vi "initializePIstages.vi"(0 "xy stage":bool=TRUE, 1 "z stage":bool=TRUE) -> (2 "XY stage":T2, 3 "Z stage":T1, 4 "current xPos (mm)":dbl, 5 "current yPos (mm)":dbl, 6 "current zPos (mm)":dbl)   [LabVIEW 2015]
panel:
  in  "Z stage":T1={"System no."=2, "zIdx"=1, "zLim (mm)"=13.0, "0, 1"=0} {"System no." min=1 step=1}
  in  "XY stage":T2={"System no."=1, "xIdx"=1, "yIdx"=2, "xLim (mm)"=67.5, "yLim (mm)"=42.5, "0, 1"=0} {"System no." min=1 step=1}
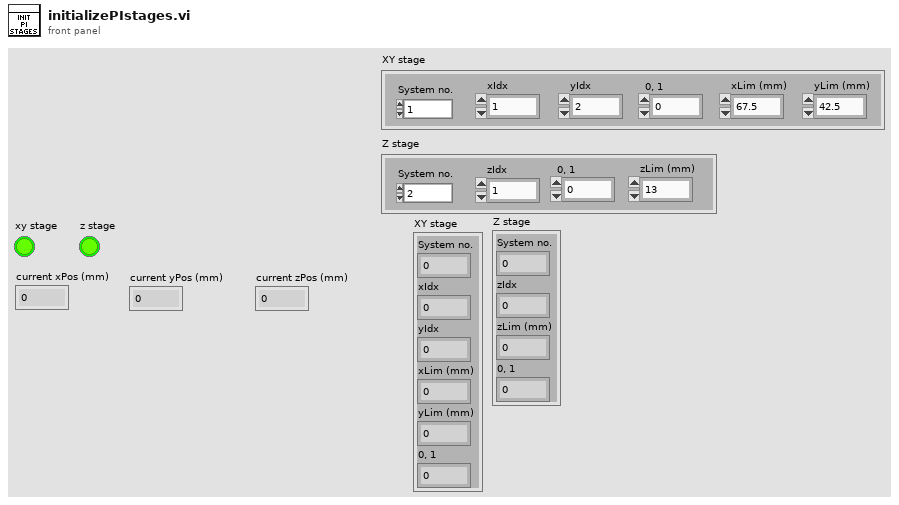
[diagram p1: front panel]
types:
  T1 = cluster{"System no.":i32, "zIdx":i32, "zLim (mm)":dbl, "0, 1":i16}
  T2 = cluster{"System no.":i32, "xIdx":i32, "yIdx":i32, "xLim (mm)":dbl, "yLim (mm)":dbl, "0, 1":i16}
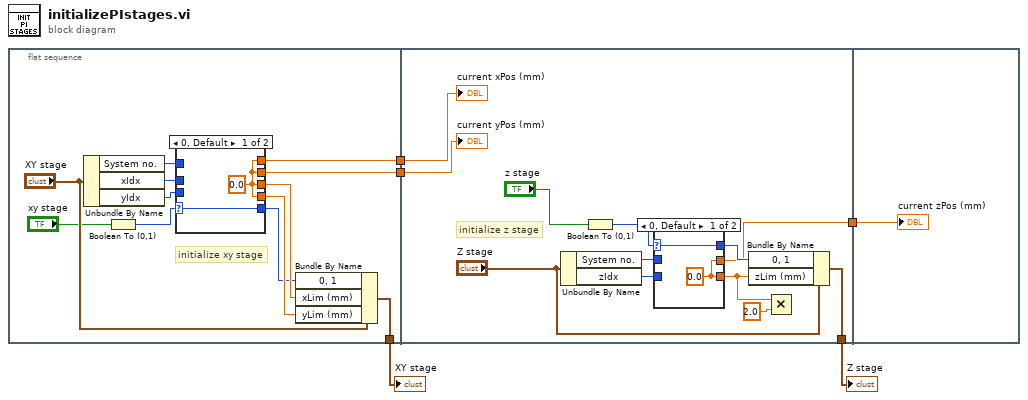
[diagram p0: block diagram]
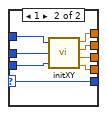
[diagram p2: hidden frame]
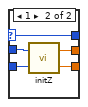
[diagram p3: hidden frame]
diagram:
  n1 = flat-sequence {
    tunnel: [w14] -> w5
    tunnel: [w13] -> w4
    tunnel: [w6] -> w2
    tunnel: w5 -> [w39]
    tunnel: w4 -> [w38]
    tunnel: [w32] -> w3
    tunnel: [w28] -> w1
    tunnel: w3 -> [w47]
    frame #0 {
      # "initialize xy stage"
      n2 = Unbundle By Name("XY stage") -> ("System no."=w17:i32, "xIdx"=w16:i32, "yIdx"=w15:i32)
      n3 = Boolean To (0,1)(Boolean="xy stage") -> (0, 1=w7:i16)
      n4 = case shown="0, Default" w7 {
        selector: w7 -> [w19 w20]
        tunnel: w17 -> [_ w27]
        tunnel: w16 -> [_ w26]
        tunnel: w15 -> [_ w25]
        tunnel: [w18 w24] -> w14
        tunnel: [w18 w23] -> w13
        tunnel: [w18 w22] -> w11
        tunnel: [w18 w21] -> w10
        tunnel: [w19 w20] -> w9
        frame 0, Default {
          w18 = 0.0 ("xPos")
        }
        frame 1 {
          n5 = call "initXY.vi"("System no."=w27, "xIdx"=w26, "yIdx"=w25) -> ("xPos"=w24:dbl, "yPos"=w23:dbl, "xLim"=w22:dbl, "yLim"=w21:dbl)
        }
      }
      n6 = Bundle By Name(cluster="XY stage", "0, 1"=w9, "xLim (mm)"=w11, "yLim (mm)"=w10) -> (w6:T2)
    }
    frame #1 {
      # "initialize z stage"
      n7 = Unbundle By Name("Z stage") -> ("System no."=w34:i32, "zIdx"=w35:i32)
      n8 = Boolean To (0,1)(Boolean="z stage") -> (0, 1=w37:i16)
      n9 = case shown="0, Default" w37 {
        selector: w37 -> [w41 w46]
        tunnel: w34 -> [_ w45]
        tunnel: w35 -> [_ w44]
        tunnel: [w41 w46] -> w36
        tunnel: [w40 w43] -> w30
        tunnel: [w40 w42] -> w32
        frame 0, Default {
          w40 = 0.0 ("xPos")
        }
        frame 1 {
          n10 = call "initZ.vi"("zIdx"=w44, "System no."=w45) -> ("zLim"=w43:dbl, "zPos"=w42:dbl)
        }
      }
      n11 = Bundle By Name(cluster="Z stage", "0, 1"=w36, "zLim (mm)"=w30) -> (w28:T1)
      n12 = Multiply(x=w30, y=2.0) -> ()  [unwired: 1 out]
      "current yPos (mm)" <- w38
      "current xPos (mm)" <- w39
    }
    frame #2 {
      "current zPos (mm)" <- w47
    }
  }
  "XY stage" <- w2
  "Z stage" <- w1
